vi "WPI_CAN_Receive.vi"(8 "error in (no error)":errorcluster, 9 "Message ID Mask":u32 format="%.0x", 10 "Message ID":u32 format="%.0x") -> (0 "error out":errorcluster, 1 "Data":u8[](array[numeric]), 2 "Message ID Out":u32 format="%.0x")   [LabVIEW 2017]
doc: "This is the low-level CAN receive VI. It may be used to communicate with generic CAN devices on the CAN bus.\n\nThis interface currently only supports receiving Extended Frames."
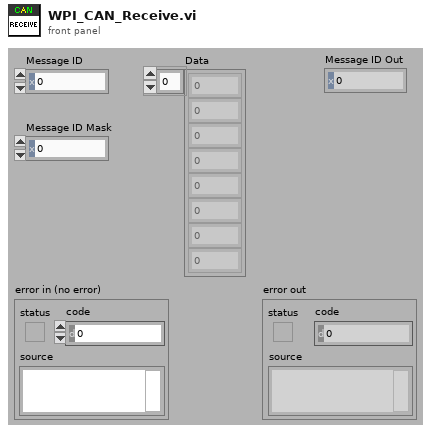
[diagram p1: front panel]
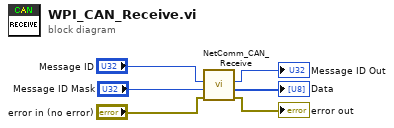
[diagram p0: block diagram]
diagram:
  n1 = call <vilib>:"NetComm_CAN_Receive.vi"("error in (no error)"="error in (no error)", "Message ID Mask"="Message ID Mask", "Message ID"="Message ID") -> ("error out"=→"error out":errorcluster, "Data"=→"Data":u8[], "Message ID Out"=→"Message ID Out":u32)  [unwired: 6 out]
